vi "Pfeiffer Vacuum Turbo Temperatur info.vi"(7 "Adress of unit":u16=1 min=1 max=999 step=1, 8 "error in (no error)":errorcluster, 9 "Parameter":T1(ring), 11 "COM Port Name in":refnum<visa-resource-name>="COM1") -> (0 "error out":errorcluster, 3 "response (data)":string)   [LabVIEW 2016]
doc: "This VI is an example of how to use the Pfeiffer Vacuum subVIs programmatically. This VI first initializes the instrument, takes measurements, then closes the instrument."
uses:
  Pfeiffer Vacuum.lvlib
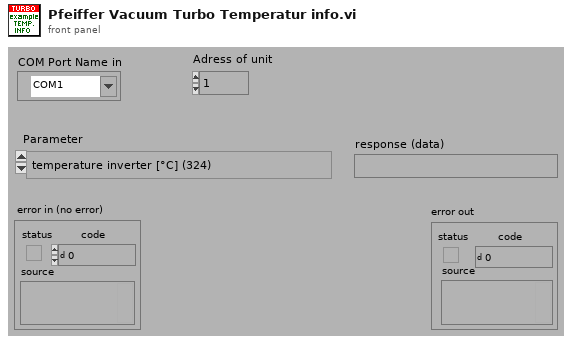
[diagram p1: front panel]
types:
  T1 = enum16{"temperature inverter [°C] (324)", "temperature electronic [°C] (326)", "temperature pump bottom [°C] (330)", "temperature bearing [°C] (342)", "temperature motor [°C] (346)"}
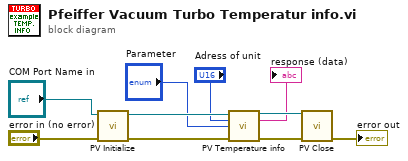
[diagram p0: block diagram]
diagram:
  n1 = call "PV Initialize.vi"("error in (no error)"="error in (no error)", "VISA session in"="COM Port Name in") -> ("error out"=w10:errorcluster, "VISA session out"=w8:refnum<visa-resource-name>)  [unwired: 8 in]
  n2 = call "PV Temperature info.vi"("VISA session"=w8, "Adress of unit"="Adress of unit", "Parameter"="Parameter", "error in (no error)"=w10) -> ("dup VISA session"=w7:refnum<visa-resource-name>, "response (data)"=→"response (data)":string, "error out"=w9:errorcluster)  [unwired: 9 in]
  n3 = call "PV Close.vi"("VISA session"=w7, "error in (no error)"=w9) -> ("error out"=→"error out":errorcluster)  [unwired: 13 in]
